vi "Main.vi"() -> ()   [LabVIEW 2015]
doc: "The myRIO Project template acquires acceleration data from the onboard accelerometer and displays the changes of acceleration values in a waveform chart."
uses:
  <vilib>/myRIO/Common/Instrument Driver Framework/myRIO v1.0/Encoder/typedefs/Encoder Signal Mode.ctl
  <vilib>/myRIO/Instrument Drivers/Onboard IO/Encoder/typedefs/Encoder Reference.ctl
  <vilib>/myRIO/Common/Instrument Driver Framework/Utilities/typedefs/myRIO Generic Hardware Reference.ctl
  <vilib>/myRIO/Common/Instrument Driver Framework/Utilities/typedefs/Hardware Version Enum.ctl
  <vilib>/myRIO/Common/Instrument Driver Framework/Utilities/typedefs/myRIO v1.0 Reference.ctl
  <vilib>/myRIO/Common/Instrument Driver Framework/Utilities/typedefs/Generic FPGA Reference.ctl
  <vilib>/myRIO/Common/Instrument Driver Framework/myRIO v1.0/Encoder/typedefs/Encoder Channels Enum.ctl
  <vilib>/myRIO/Common/Instrument Driver Framework/myRIO v1.0/Encoder/typedefs/Encoder Configuration v1.0.ctl
  <vilib>/userdefined/High Color/nirio_resource_hc.ctl
  <vilib>/myRIO/Instrument Drivers/Onboard IO/DIO/typedefs/DIO Reference.ctl
  <vilib>/myRIO/Common/Instrument Driver Framework/myRIO v1.0/DIO/typedefs/DIO Channels List.ctl
  <vilib>/myRIO/Common/Instrument Driver Framework/myRIO v1.0/DIO/typedefs/DIO Channels Enum.ctl
  <vilib>/myRIO/Instrument Drivers/Onboard IO/PWM/typedefs/PWM Reference.ctl
  <vilib>/myRIO/Common/Instrument Driver Framework/myRIO v1.0/PWM/typedefs/PWM Channels Enum.ctl
  <vilib>/myRIO/Instrument Drivers/Onboard IO/PWM/typedefs/PWM Configuration.ctl
  <vilib>/myRIO/Common/Instrument Driver Framework/Utilities/vis/Is FPGA Ref Available.vi
  <vilib>/myRIO/Common/Instrument Driver Framework/myRIO v1.0/Encoder/vis/myRIO v1.1 Open Encoder.vi
  <vilib>/myRIO/Instrument Drivers/Onboard IO/Encoder/vis/Read.vi
  <vilib>/myRIO/Common/Instrument Driver Framework/myRIO v1.0/DIO/vis/myRIO v1.1 Open DIO.vi
  <vilib>/myRIO/Instrument Drivers/Onboard IO/DIO/vis/Write.vi
  <vilib>/myRIO/Common/Instrument Driver Framework/myRIO v1.0/PWM/vis/myRIO v1.1 Open PWM.vi
  <vilib>/myRIO/Instrument Drivers/Onboard IO/PWM/vis/Set Duty Cycle and Frequency.vi
  <vilib>/myRIO/Common/Instrument Driver Framework/Utilities/vis/Validate Channels.vi
  <vilib>/myRIO/Common/Instrument Driver Framework/myRIO v1.0/Encoder/vis/myRIO v1.0 Reserve Encoder.vi
  <vilib>/myRIO/Common/Instrument Driver Framework/myRIO v1.0/DIO/vis/myRIO v1.0 Reserve DIO.vi
  <vilib>/myRIO/Common/Instrument Driver Framework/myRIO v1.0/PWM/vis/myRIO v1.0 Reserve PWM.vi
  <vilib>/myRIO/Common/Instrument Driver Framework/myRIO v1.0/UART/vis/myRIO v1.0 Close UART.vi
  <vilib>/myRIO/Common/Instrument Driver Framework/myRIO v1.0/Encoder/vis/myRIO v1.0 Build MUX Configuration Encoder.vi
  <vilib>/myRIO/Common/Instrument Driver Framework/myRIO v1.0/Resource Manager/vis/myRIO v1.0 Reserve Channel List.vi
  <vilib>/myRIO/Common/Instrument Driver Framework/myRIO v1.0/DIO/vis/myRIO v1.0 Build MUX Configuration DIO.vi
  <vilib>/myRIO/Common/Instrument Driver Framework/myRIO v1.0/PWM/vis/myRIO v1.0 Build MUX Configuration PWM.vi
  <vilib>/myRIO/Common/Instrument Driver Framework/myRIO v1.0/Resource Manager/vis/myRIO v1.0 Create Configuration List.vi
  <vilib>/myRIO/Common/Instrument Driver Framework/myRIO v1.0/Resource Manager/vis/myRIO v1.0 Reserve Channel.vi
  <vilib>/myRIO/Common/Instrument Driver Framework/myRIO v1.0/Resource Manager/vis/myRIO v1.0 Unreserve Channel.vi
  <vilib>/myRIO/Common/Instrument Driver Framework/myRIO v1.0/Resource Manager/vis/myRIO v1.0 Build Mutex Name.vi
  <vilib>/Utility/VariantDataType/GetNumericInfo.vi
  <vilib>/Utility/error.llb/Error Cluster From Error Code.vi
  <vilib>/myRIO/Common/Instrument Driver Framework/myRIO v1.0/myRIO v1.1 Open.vi
  <vilib>/myRIO/Common/Instrument Driver Framework/Utilities/vis/IO Manager.vi
  <vilib>/myRIO/Common/Instrument Driver Framework/Utilities/vis/Configuration Manager.vi
  <vilib>/myRIO/Common/Instrument Driver Framework/myRIO v1.0/Resource Manager/vis/myRIO v1.0 Configure IO.vi
  <vilib>/myRIO/Common/Instrument Driver Framework/myRIO v1.0/myRIO v1.0 Close.vi
  <vilib>/myRIO/Common/Instrument Driver Framework/myRIO v1.0/Encoder/vis/myRIO v1.0 Configure Encoder.vi
  <vilib>/myRIO/Common/Instrument Driver Framework/myRIO v1.0/Encoder/vis/myRIO v1.0 Read Encoder.vi
  <vilib>/myRIO/Common/Instrument Driver Framework/myRIO v1.0/DIO/vis/myRIO v1.0 Write DIO.vi
  <vilib>/myRIO/Common/Instrument Driver Framework/myRIO v1.0/PWM/vis/myRIO v1.0 Write PWM.vi
  <vilib>/myRIO/Common/Instrument Driver Framework/Utilities/vis/FPGA Ref Manager.vi
  <vilib>/myRIO/Common/Instrument Driver Framework/myRIO v1.0/myRIO v1.0 Reset FPGA.vi
  <vilib>/myRIO/Common/Instrument Driver Framework/myRIO v1.0/IRQ/vis/myRIO v1.0 IRQ Info FGV.vi
  <vilib>/myRIO/Common/Instrument Driver Framework/myRIO v1.0/IRQ/vis/myRIO v1.0 Timer IRQ Info FGV.vi
  <vilib>/myRIO/Common/Instrument Driver Framework/myRIO v1.0/IRQ/vis/myRIO v1.0 ISR Agent.vi
  <vilib>/myRIO/Express VI/Onboard IO/Encoder/Encoder Express VI.xnode
  <vilib>/myRIO/Common/Instrument Driver Framework/myRIO v1.0/Encoder/typedefs/Encoder Count Direction Enum.ctl
  <vilib>/myRIO/Instrument Drivers/Onboard IO/Encoder/vis/myRIO Encoder Open.xnode
  <vilib>/myRIO/Express VI/Onboard IO/DO/DO Express VI.xnode
  <vilib>/myRIO/Instrument Drivers/Onboard IO/DIO/vis/myRIO DIO Open.xnode
  <vilib>/myRIO/Express VI/Onboard IO/PWM/PWM Express VI.xnode
  <vilib>/myRIO/Instrument Drivers/Onboard IO/PWM/vis/myRIO PWM Open.xnode
  <vilib>/myRIO/Instrument Drivers/Utilities/Utilities.lvlib
  <vilib>/myRIO/Instrument Drivers/Onboard IO/Encoder/Encoder.lvlib
  <vilib>/myRIO/Instrument Drivers/Onboard IO/DIO/DIO.lvlib
  <vilib>/myRIO/Instrument Drivers/Onboard IO/PWM/PWM.lvlib
panel:
  out "Waveform Chart 4":dbl(graph)
  in  "ON OFF":bool
  out "x >= 0?":bool
  out ".not. x?":bool
  out "abs(x)":dbl
  out "filtTheta":dbl
  out "Theta control 2":dbl
  out "Waveform Chart":dbl(graph)
  out "Theta control":dbl
  out "Control":bool
  out "dPhi":dbl(graph)
  out "dTheta":dbl(graph)
  in  "Swing up gain":dbl
  out "Rad dTheta":dbl
  out "Rad dPhi":dbl
  out "Rad Theta":dbl
  out "Rad Phi":dbl
  out "Direction Motor":dbl
  out "Counter Motor":dbl
  in  "Stop Button":bool
  out "error out":errorcluster
  # "Overview: The myRIO Project template acquires acceleration data from the onboard accelerometer and displays the changes of acceleration values in a waveform chart.\nInstructions:\n1. Check the myRIO target IP address in the project and make sure the target IP address is correct. \n2. Run this VI."
types:
  T1 = typedef "Encoder.lvlib/Encoder Reference.ctl" = cluster{"myRIO Reference":T2, "Encoder Channels Enum":T6}
  T2 = typedef "myRIO Generic Hardware Reference.ctl" = cluster{"myRIO Model":T3, "myRIO Hardware Reference":T4}
  T3 = typedef "Hardware Version Enum.ctl" = enum16{"Unknown", "myRIO-1900", "myRIO-1950", "roboRIO"}
  T4 = typedef "myRIO v1.0 Reference.ctl" = cluster{"Generic FPGA Reference":T5, "Allow multiple opens":bool}
  T5 = typedef "Generic FPGA Reference.ctl" = refnum<k20>
  T6 = typedef "Encoder Channels Enum.ctl" = enum16{"Not Connected", "C/ENC0", "C/ENC1", "A/ENC", "B/ENC", "DIO/ENC0", "DIO/ENC1", "DIO/ENC2", "DIO/ENC3", "DIO/ENC4"}
  T7 = typedef "Encoder Signal Mode.ctl" = enum16{"Quadrature phase signal", "Step and direction signal"}
  T8 = typedef "nirio_resource_hc.ctl" = tag
  T9 = typedef "DIO.lvlib/DIO Reference.ctl" = cluster{"myRIO Reference":T2, "DIO Channels List":T10}
  T10 = typedef "DIO Channels List.ctl" = T11[]
  T11 = typedef "DIO Channels Enum.ctl" = enum16{"Not Connected", "C/DIO0", "C/DIO1", "C/DIO2", "C/DIO3", "C/DIO4", "C/DIO5", "C/DIO6", "C/DIO7", "A/DIO0", "A/DIO1", "A/DIO2", "A/DIO3", "A/DIO4", "A/DIO5", "A/DIO6", "A/DIO7", "A/DIO8", "A/DIO9", "A/DIO10", "A/DIO11", "A/DIO12", "A/DIO13", "A/DIO14", "A/DIO15", "B/DIO0", "B/DIO1", "B/DIO2", "B/DIO3", "B/DIO4", "B/DIO5", "B/DIO6", "B/DIO7", "B/DIO8", "B/DIO9", "B/DIO10", "B/DIO11", "B/DIO12", "B/DIO13", "B/DIO14", "B/DIO15", "LED0", "LED1", "LED2", "LED3", "Button0", "DIO/DIO0", "DIO/DIO1", "DIO/DIO2", "DIO/DIO3", "DIO/DIO4", "DIO/DIO5", "DIO/DIO6", "DIO/DIO7", "DIO/DIO8", "DIO/DIO9", "SPI/CS0", "SPI/CS1", "SPI/CS2", "SPI/CS3", "LED RADIO (Green)", "LED RADIO (Red)", "LED COMM (Green)", "LED COMM (Red)", "LED MODE (Green)", "LED MODE (Red)"}
  T12 = typedef "PWM.lvlib/PWM Reference.ctl" = cluster{"myRIO Reference":T2, "PWM Channels Enum":T13, "PWM Configuration":T14}
  T13 = typedef "PWM Channels Enum.ctl" = enum16{"Not Connected", "C/PWM0", "C/PWM1", "A/PWM0", "A/PWM1", "A/PWM2", "B/PWM0", "B/PWM1", "B/PWM2", "PWM/PWM0", "PWM/PWM1", "PWM/PWM2", "PWM/PWM3", "PWM/PWM4", "PWM/PWM5", "PWM/PWM6", "PWM/PWM7", "PWM/PWM8", "PWM/PWM9"}
  T14 = typedef "PWM.lvlib/PWM Configuration.ctl" = cluster{"Frequency":dbl, "Duty Cycle":dbl}
  T15 = typedef "Encoder Count Direction Enum.ctl" = enum16{"Counting Up", "Counting Down"}
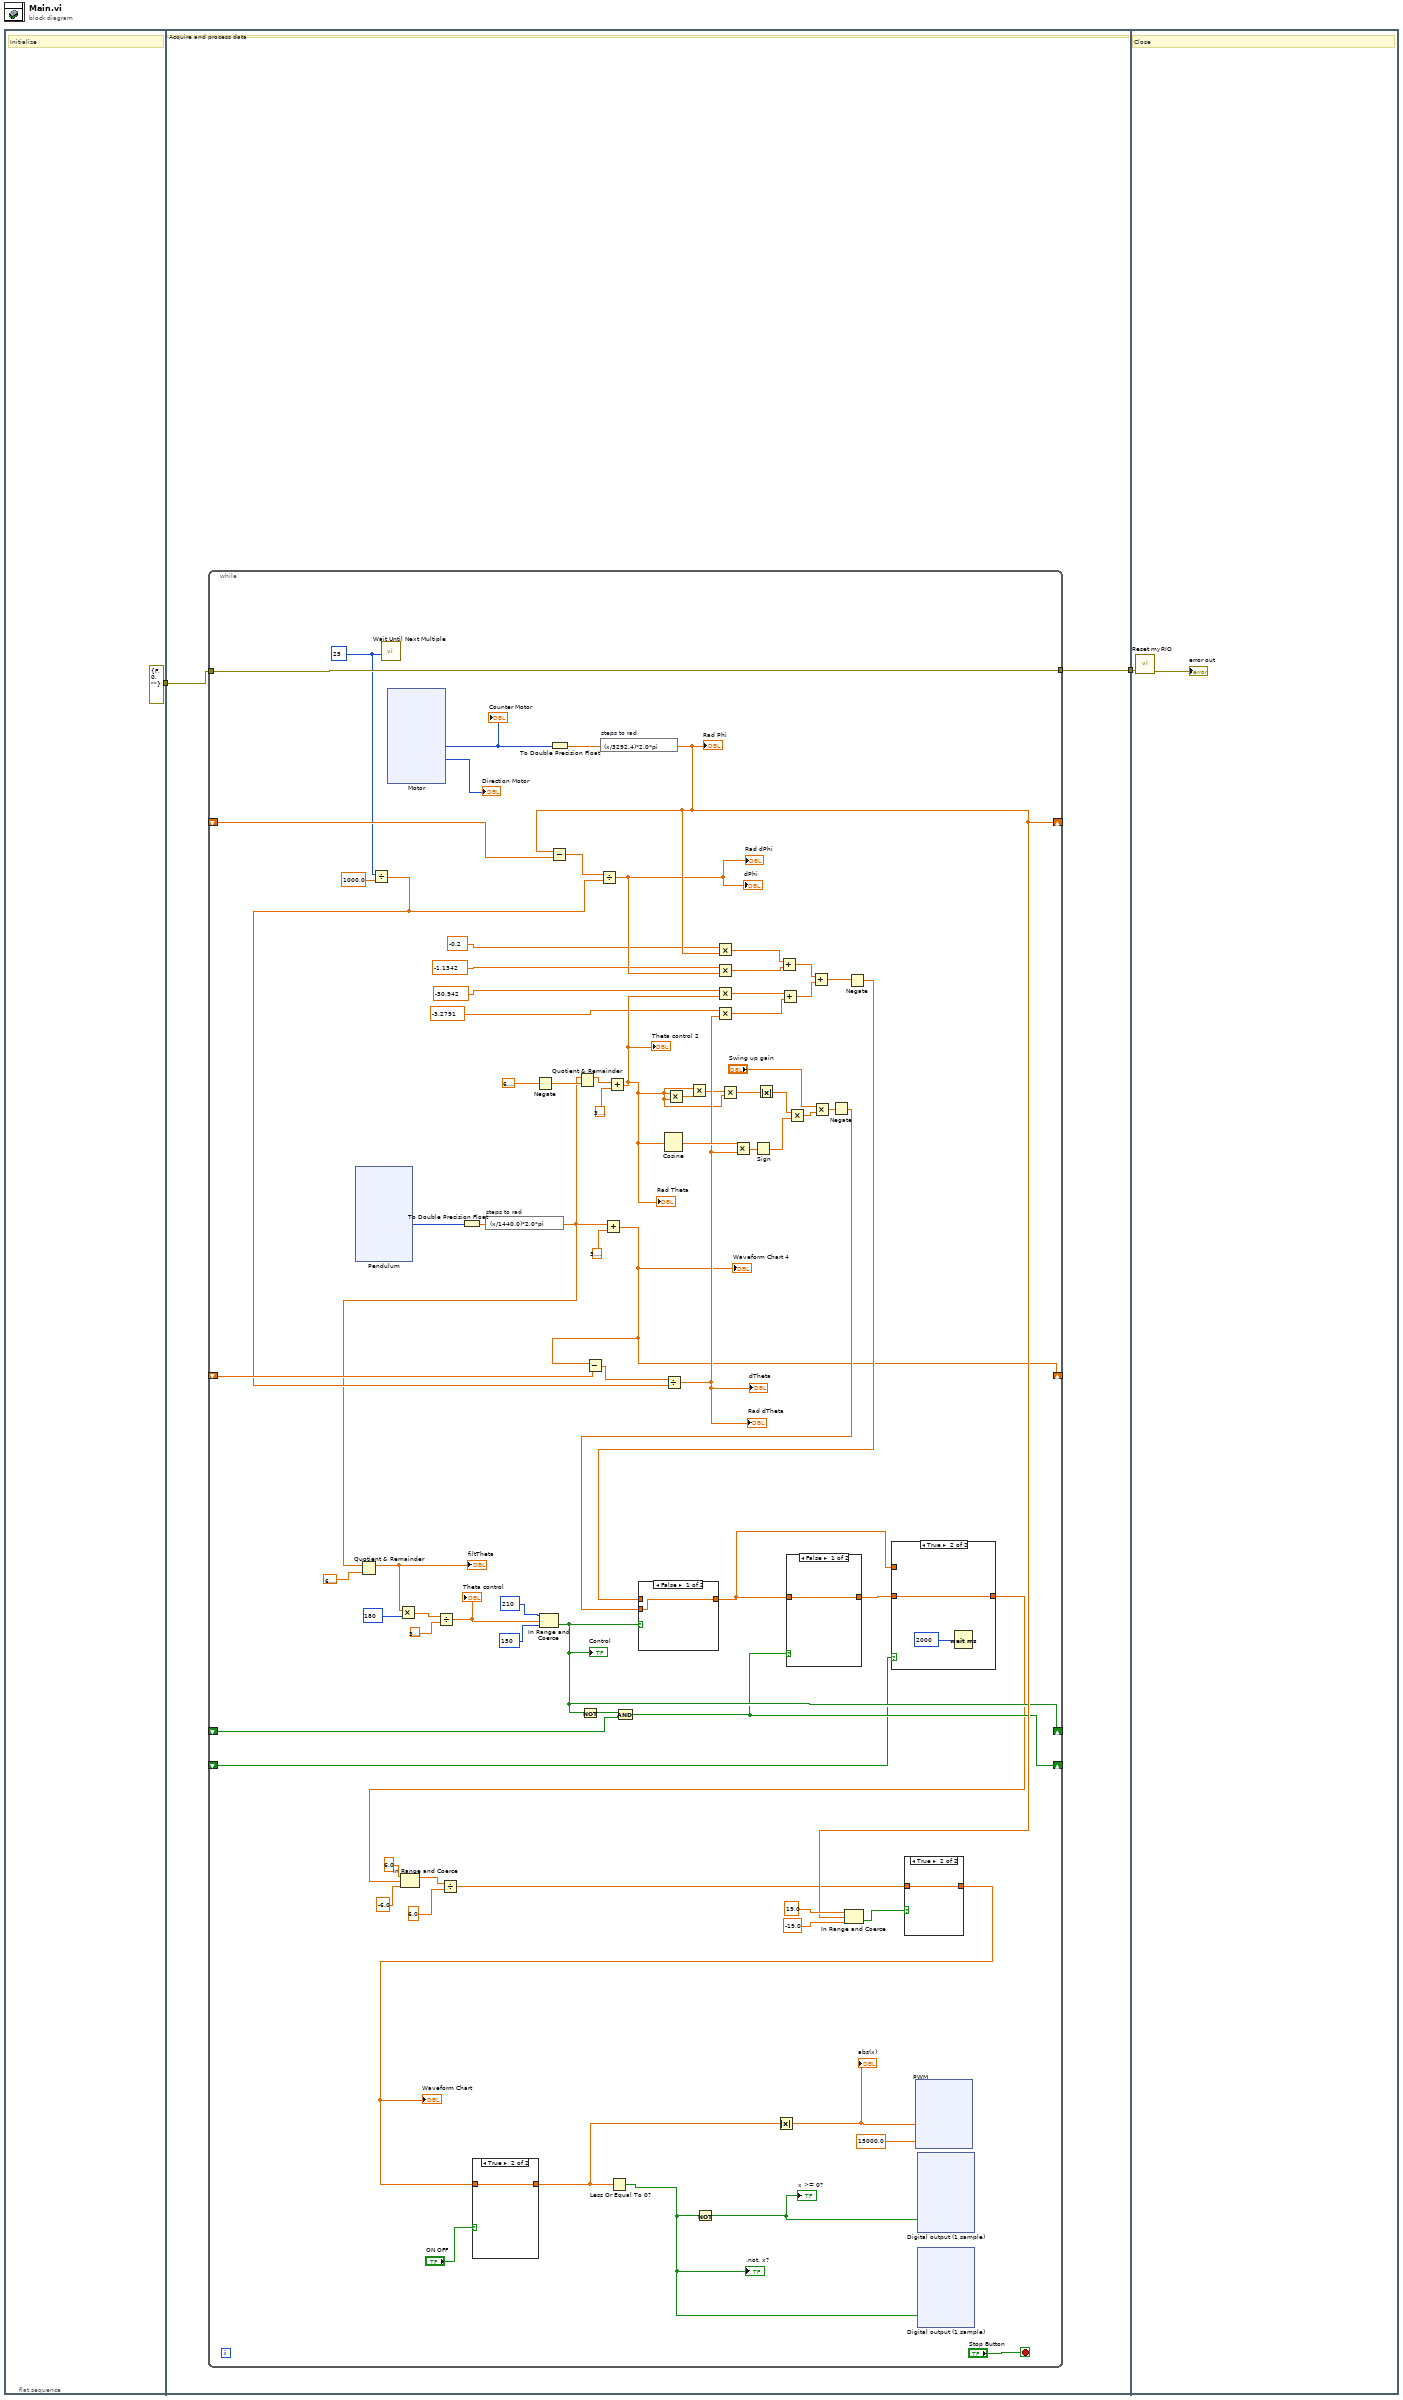
[diagram p0: block diagram]
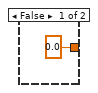
[diagram p2: hidden frame]
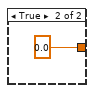
[diagram p4: hidden frame]
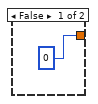
[diagram p6: hidden frame]
diagram:
  n1 = flat-sequence {
    tunnel: [errorcluster {"status"=FALSE, "code"=0, "source"=""} ("error in (no error)")] -> w2
    tunnel: w2 -> [w4]
    tunnel: [w5] -> w1
    tunnel: w1 -> [w294]
    frame #0 {
      # "Initialize"
    }
    frame #1 {
      # "Acquire and process data"
      n2 = while {
        tunnel: w4 -> [w79]
        tunnel: [w79] -> w5
        shift-right: [w62] -> _
        shift-left: _ -> [w78]
        shift-right: [w10] -> _
        shift-left: _ -> [w75]
        shift-right: [w24] -> _
        shift-left: _ -> [w23]
        shift-right: [w22] -> _
        shift-left: _ -> [w21]
        stop <- "Stop Button" stop-if-true
        w27 = u32 25 ("Count(mSec)")
        n3 = xnode "Pendulum"() -> ("Counter Value"=w7:i32)  [unwired: 2 in, 3 out]
        n4 = Divide(x=w27, y=1000.0) -> (x/y=w26:dbl)
        n5 = call "Wait Until Next Multiple"("Count(mSec)"=w27) -> ()  [unwired: 1 out]
        n6 = xnode "Motor"() -> ("Counter Value"=w83:i32, "Counter Direction"=→"Direction Motor":T15)  [unwired: 2 in, 2 out]
        "Counter Motor" <- w83
        n7 = To Double Precision Float(number=w7) -> (double precision float=w82:dbl)
        n8 = expression code="(x/1440.0)*2.0*pi" "steps to rad"(w82) -> (w9:dbl)
        n9 = Quotient & Remainder(x=w9, y=6.283185307179586) -> (x-y*floor(x/y)=w52:dbl)  [unwired: 1 out]
        "filtTheta" <- w52
        n10 = Multiply(x=w52, y=180) -> (x*y=w50:dbl)
        n11 = Divide(x=w50, y=3.141592653589793) -> (x/y=w8:dbl)
        "Theta control" <- w8
        n12 = Negate(x=6.283185307179586) -> (-x=w37:dbl)
        n13 = In Range and Coerce(upper limit=210, x=w8, lower limit=150) -> (In Range?=w24:bool)  [unwired: 1 out]
        "Control" <- w24
        n14 = To Double Precision Float(number=w83) -> (double precision float=w81:dbl)
        n15 = Quotient & Remainder(x=w9, y=w37) -> (x-y*floor(x/y)=w38:dbl)  [unwired: 1 out]
        n16 = Not(x=w24) -> (.not. x?=w25:bool)
        n17 = expression code="(x/3292.4)*2.0*pi" "steps to rad"(w81) -> (w62:dbl)
        "Rad Phi" <- w62
        n18 = Subtract(x=w62, y=w78) -> (x-y=w77:dbl)
        n19 = Divide(x=w77, y=w26) -> (x/y=w61:dbl)
        "Rad dPhi" <- w61
        "dPhi" <- w61
        n20 = Add(x=w9, y=3.141592653589793) -> (x+y=w10:dbl)
        "Waveform Chart 4" <- w10
        n21 = Subtract(x=w10, y=w75) -> (x-y=w76:dbl)
        n22 = Add(x=w38, y=3.141592653589793) -> (x+y=w35:dbl)
        "Rad Theta" <- w35
        "Theta control 2" <- w35
        n23 = And(x=w25, y=w23) -> (x .and. y?=w22:bool)
        n24 = Cosine(x=w35) -> (cos(x)=w73:dbl)
        n25 = Divide(x=w76, y=w26) -> (x/y=w60:dbl)
        "Rad dTheta" <- w60
        "dTheta" <- w60
        n26 = Multiply(x=w35, y=w35) -> (x*y=w66:dbl)
        n27 = Multiply(x=w35, y=w66) -> (x*y=w36:dbl)
        n28 = Multiply(x=-0.2 ("element"), y=w62) -> (x*y=w54:dbl)
        n29 = Multiply(x=-1.1342 ("element"), y=w61) -> (x*y=w55:dbl)
        n30 = Multiply(x=-30.942 ("element"), y=w35) -> (x*y=w56:dbl)
        n31 = Multiply(x=-3.2791 ("element"), y=w60) -> (x*y=w57:dbl)
        n32 = Multiply(x=w36, y=w35) -> (x*y=w34:dbl)
        n33 = Multiply(x=w73, y=w60) -> (x*y=w72:dbl)
        n34 = Sign(1:w72) -> (0:w74:dbl)
        n35 = Absolute Value(x=w34) -> (abs(x)=w67:dbl)
        n36 = Add(x=w54, y=w55) -> (x+y=w59:dbl)
        n37 = Add(x=w56, y=w57) -> (x+y=w58:dbl)
        n38 = Multiply(x=w67, y=w74) -> (x*y=w65:dbl)
        n39 = Add(x=w59, y=w58) -> (x+y=w46:dbl)
        n40 = Multiply(x="Swing up gain", y=w65) -> (x*y=w53:dbl)
        n41 = Negate(x=w53) -> (-x=w17:dbl)
        n42 = In Range and Coerce(upper limit=19.0, x=w62, lower limit=-19.0 ("upper limit")) -> (In Range?=w68:bool)  [unwired: 1 out]
        n43 = Negate(x=w46) -> (-x=w41:dbl)
        n44 = case shown="False" w24 {
          tunnel: w41 -> [_ w209]
          tunnel: w17 -> [w208 _]
          tunnel: [w208 w209] -> w18
          frame False {
          }
          frame True {
          }
        }
        n45 = case shown="False" w22 {
          tunnel: w18 -> [w206 _]
          tunnel: [w206 0.0] -> w20
          frame False {
          }
          frame True {
          }
        }
        n46 = case shown="True" w21 {
          tunnel: w20 -> [_ w204]
          tunnel: [w203 w204] -> w19
          tunnel: w18 -> [w203 _]
          frame False {
          }
          frame True {
            n47 = Wait (ms)(milliseconds to wait=u32 2000) -> ()  [unwired: 1 out]
          }
        }
        n48 = In Range and Coerce(upper limit=6.0, x=w19, lower limit=-6.0) -> (coerced(x)=w42:dbl)  [unwired: 1 out]
        n49 = Divide(x=w42, y=6.0) -> (x/y=w33:dbl)
        n50 = case shown="True" w68 {
          tunnel: [0 w211] -> w12
          tunnel: w33 -> [_ w211]
          frame False {
          }
          frame True {
          }
        }
        "Waveform Chart" <- w12
        n51 = case shown="True" "ON OFF" {
          tunnel: [0.0 w132] -> w13
          tunnel: w12 -> [_ w132]
          frame False {
          }
          frame True {
          }
        }
        n52 = Less Or Equal To 0?(x=w13) -> (x <= 0?=w15:bool)
        ".not. x?" <- w15
        n53 = Not(x=w15) -> (.not. x?=w16:bool)
        "x >= 0?" <- w16
        n54 = Absolute Value(x=w13) -> (abs(x)=w6:dbl)
        "abs(x)" <- w6
        n55 = xnode "PWM"("Duty Cycle"=w6, "Frequency [Hz]"=15000.0) -> ()  [unwired: 1 in, 1 out]
        n56 = xnode "Digital output (1 sample)"("A/DIO8 (Pin 27)"=w16) -> ()  [unwired: 1 in, 1 out]
        n57 = xnode "Digital output (1 sample)"("A/DIO9 (Pin 29)"=w15) -> ()  [unwired: 1 in, 1 out]
      }
    }
    frame #2 {
      # "Close"
      n58 = call <vilib>:"Reset myRIO.vi"("error in (no error)"=w294) -> ("error out"=→"error out":errorcluster)  [unwired: 10 in]
    }
  }
